vi "Error Handler.vi"(8 "error in (no error)":errorcluster, 11 "View Model":T1) -> (0 "error out":errorcluster, 3 "View Model":T1)   [LabVIEW 2017]
doc: "Defines and handles all levels of Car Wash Errors."
uses:
  View Model/Controls/View Model.ctl
  View Model/Controls/Shared Model.ctl
  Controls/Error Model.ctl
  Controls/Error Data.ctl
  Controls/Error Level.ctl
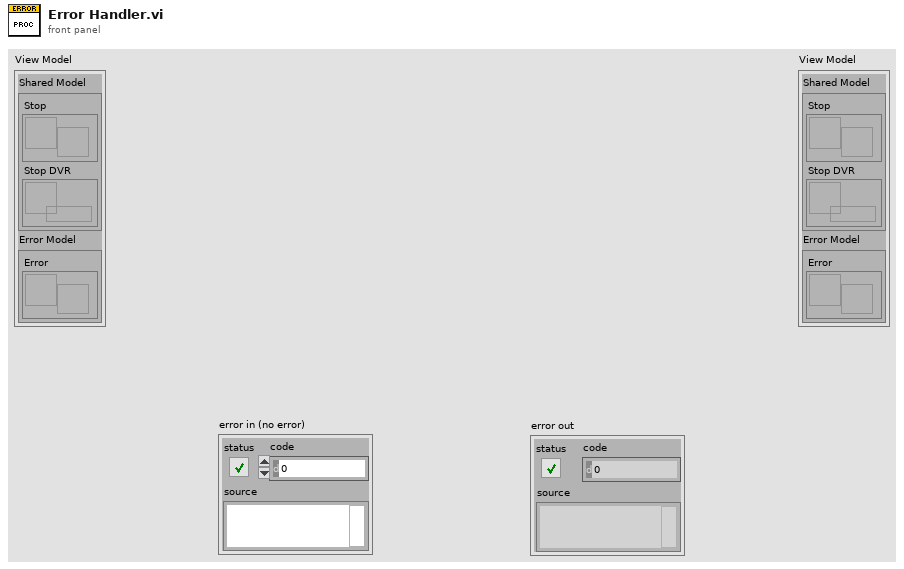
[diagram p1: front panel]
types:
  T1 = typedef "View Model.ctl" = cluster{"Shared Model":T2, "Error Model":T3}
  T2 = typedef "Shared Model.ctl" = cluster{"Stop":refnum<user-event>, "Stop DVR":refnum<data-value>}
  T3 = typedef "Error Model.ctl" = cluster{"Error":refnum<user-event>}
  T4 = typedef "Error Level.ctl" = enum16{"Minor Error", "Wash Cycle Error", "System Error"}
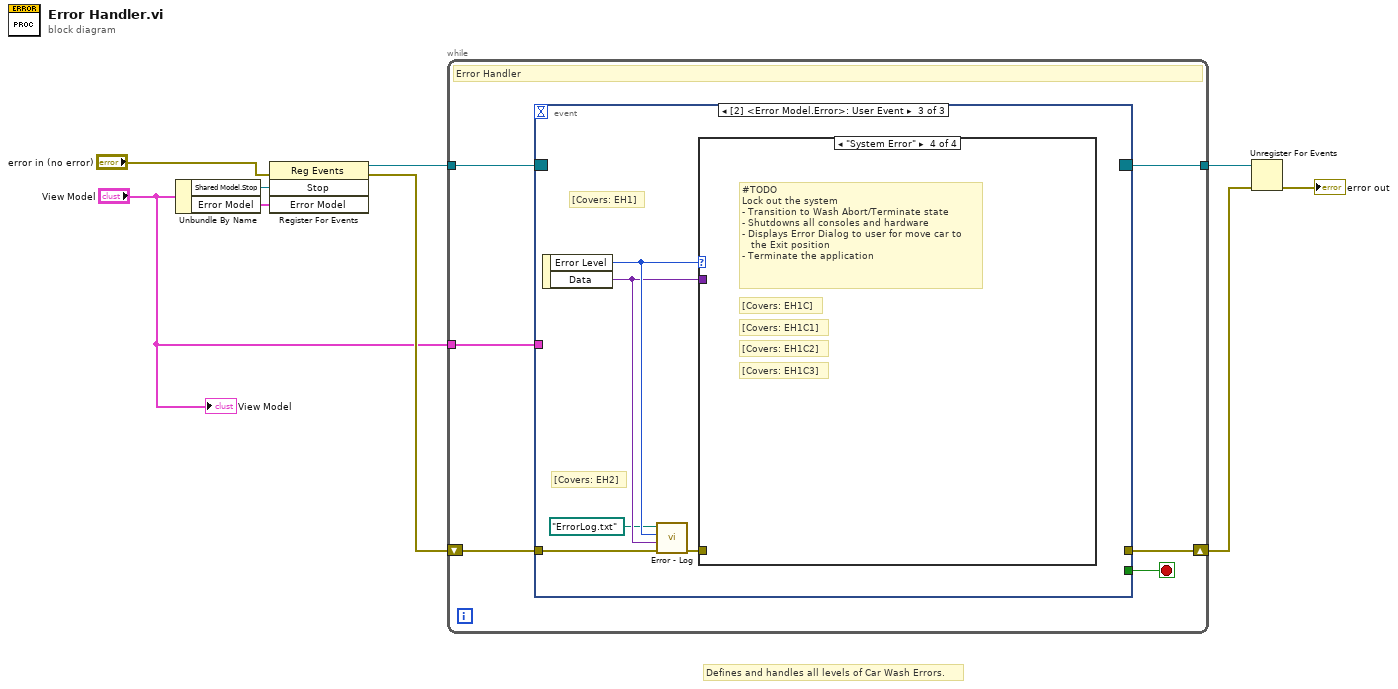
[diagram p0: block diagram]
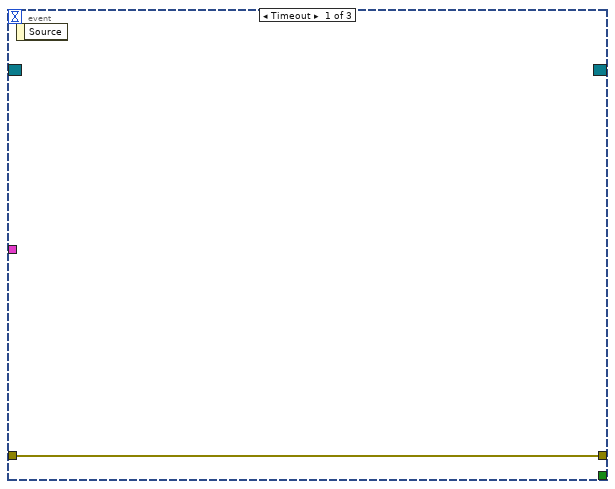
[diagram p2: hidden frame]
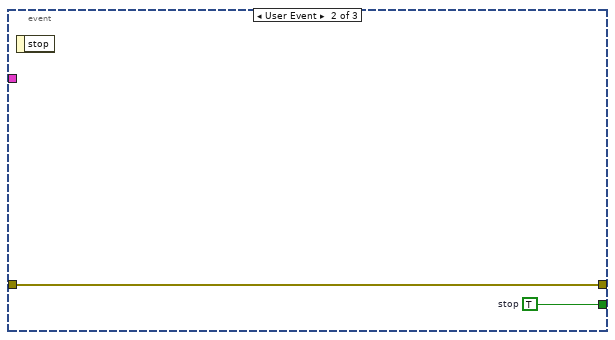
[diagram p3: hidden frame]
diagram:
  # "Defines and handles all levels of Car Wash Errors."
  n1 = Unbundle By Name("View Model") -> ("Shared Model.Stop"=w9:refnum<user-event>, "Error Model"=w1:T3)
  n2 = register-events(error in="error in (no error)", w9, w1) -> (reference out=w7:refnum<event-registration>, error out=w6:errorcluster)  [unwired: 1 in]
  n3 = while {
    tunnel: w7 -> [w15]
    shift-right: [w13] -> w4
    shift-left: w6 -> [w14]
    tunnel: [w11] -> w5
    tunnel: "View Model" -> [w10]
    stop <- w12 stop-if-true
    # "Error Handler"
    n4 = event shown="[2] <Error Model.Error>: User Event" {
      selector: w15 -> [_ _ _]
      dyn-events: [_ _ _] -> w11
      timeout: _ -> [_ _ _]
      tunnel: w14 -> [w16 w18 w23]
      tunnel: [w16 w18 _] -> w13
      tunnel: [_ w17 _] -> w12
      tunnel: w10 -> [_ _ _]
      event Timeout {
        n5 = event-data() -> ()  [unwired: 1 in, 1 out]
      }
      event User Event {
        w17 = TRUE  # stop
        n6 = event-data() -> ()  [unwired: 1 in, 1 out]
      }
      event User Event {
        # "[Covers: EH1]"
        # "[Covers: EH2]"
        n7 = event-data() -> ("Error Level"=w22:T4, "Data"=w21:variant)  [unwired: 1 in]
        n8 = call "Error - Log.vi"("error in (no error)"=w23, "Data"=w21, "Error Level"=w22, "Error Log Path"=path "ErrorLog.txt") -> ("error out"=w19:errorcluster)  [unwired: 7 in]
        n9 = case shown="\"System Error\"" w22 {
          tunnel: w21 -> [_ _ _ _]
          tunnel: w19 -> [_ _ _ _]
          frame Default {
            # "#TODO\nProcessing not specified error level"
          }
          frame "Minor Error" {
            # "[Covers: EH1A]"
            # "#TODO\nContinue operations without any user interuption."
          }
          frame "Wash Cycle Error" {
            # "[Covers: EH1B2]"
            # "[Covers: EH1B1]"
            # "[Covers: EH1B]"
            # "#TODO\n-Transition to Wash Abort/Terminate state.\n- Displays Error Dialog to the user for move car\n  to the Exit position.\n- Reinit Car Wash controller for new Wash cycle"
          }
          frame "System Error" {
            # "[Covers: EH1C3]"
            # "[Covers: EH1C2]"
            # "[Covers: EH1C1]"
            # "[Covers: EH1C]"
            # "#TODO\nLock out the system\n- Transition to Wash Abort/Terminate state\n- Shutdowns all consoles and hardware\n- Displays Error Dialog to user for move car to\n   the Exit position\n- Terminate the application"
          }
        }
      }
    }
  }
  n10 = Unregister For Events(event registration refnum=w5, error in=w4) -> (error out=→"error out":errorcluster)
  "View Model" <- "View Model"
